vi "Open ColorProcessorSDK.vi"(8 "error in (no error)":errorcluster) -> (0 "error out":errorcluster, 3 "ColorProcessorSDK reference":refnum<k24>)   [LabVIEW 2015]
uses:
  C:/code/ScientificCameraInterfaces/Installer/Scientific Camera Interfaces/LabVIEW/64_bit/Library_X64/Thorlabs.TSI.ColorProcessor.dll
  code/ScientificCameraInterfaces/Installer/Scientific Camera Interfaces/LabVIEW/64_bit/Library_X64/Thorlabs.TSI.ColorProcessor.dll
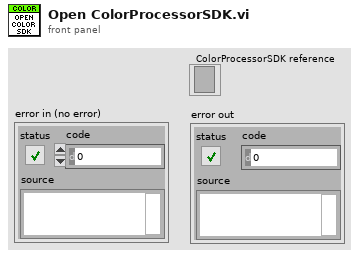
[diagram p1: front panel]
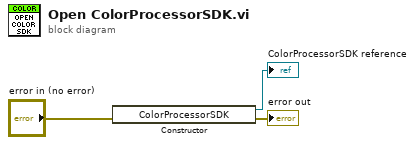
[diagram p0: block diagram]
diagram:
  n1 = constructor class="ColorProcessorSDK"(error in="error in (no error)") -> (reference out=→"ColorProcessorSDK reference":refnum<k24>, error out=→"error out":errorcluster)  [unwired: 2 in, 1 out]
